vi "GPS PositionChange Event Example.vi"() -> ()   [LabVIEW 2012, in "Phidget GPS.lvlib"]
uses:
  <instrlib>/Phidgets/Phidget GPS/Phidget GPS.lvlib
  <instrlib>/Phidgets/Phidget GPS/Public/GPSStart.vi
  <instrlib>/Phidgets/Phidget GPS/Public/GPSClose.vi
  <instrlib>/Phidgets/Phidget Common/Phidget Common.lvlib
panel:
  out "Latitude":dbl
  out "Longitude":dbl
  out "Altitude":dbl
  in  "stop":bool
  out "Serial Number Return":i32
  in  "Device Info":T1={"Serial Number"=-1, "Channel"=0, "Port"=0}
  out "error out":errorcluster
  # "Be sure to use this stop button to stop the program.\nIf you use the \"Abort Execution\" button, you will\nneed to use PhidgetResetLibrary.vi or restart Labview \nin order for any Phidgets to work."
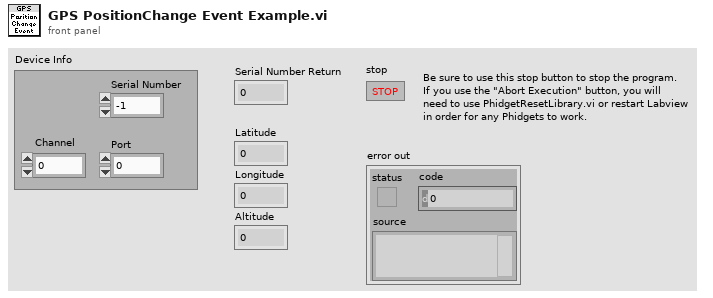
[diagram p1: front panel]
types:
  T1 = cluster{"Serial Number":i32, "Channel":i32, "Port":i32}
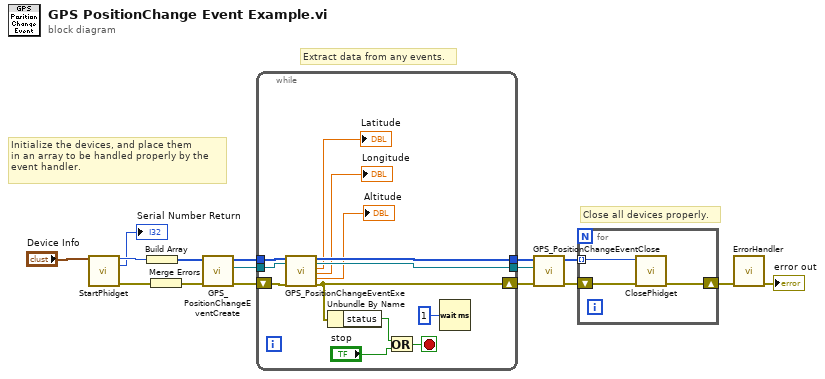
[diagram p0: block diagram]
diagram:
  # "Close all devices properly."
  # "Extract data from any events."
  # "Initialize the devices, and place them\nin an array to be handled properly by the\nevent handler."
  n1 = call-poly <instrlib>:"StartPhidget.vi"("Device Info"="Device Info") -> ("Phidget ID"=w5:u64, "Serial Number Return"=→"Serial Number Return":i32, "error out"=w1:errorcluster)  [unwired: 11 in, 1 out]
  n2 = Build Array(w5) -> (w16:u64[])
  n3 = Merge Errors(w1) -> (w7:errorcluster)
  n4 = call <instrlib>:"GPS_PositionChangeEventCreate.vi"("error in (no error)"=w7, "Devices In"=w16) -> ("error out"=w9:errorcluster, "Event Registration Refnum"=w14:refnum<event-registration>, "Devices Out"=w15:u64[])  [unwired: 7 in]
  n5 = while {
    tunnel: w15 -> [w29]
    tunnel: w14 -> [w24]
    tunnel: [w28] -> w11
    shift-right: [w23] -> w10
    shift-left: w9 -> [w27]
    tunnel: [w25] -> w3
    stop <- w22 stop-if-true
    n6 = call <instrlib>:"GPS_PositionChangeEventExe.vi"("Devices In"=w29, "Event Registration Refnum In"=w24, "error in (no error)"=w27) -> ("Devices Out"=w25:u64[], "Event Registration Refnum Out"=w28:refnum<event-registration>, "Latitude"=→"Latitude":dbl, "Longitude"=→"Longitude":dbl, "Altitude"=→"Altitude":dbl, "error out"=w23:errorcluster)  [unwired: 8 in, 3 out]
    n7 = Unbundle By Name(w23) -> ("status"=w20:bool)
    n8 = Or(x=w20, y="stop") -> (x .or. y?=w22:bool)
    n9 = Wait (ms)(milliseconds to wait=u32 1) -> ()  [unwired: 1 out]
  }
  n10 = call <instrlib>:"GPS_PositionChangeEventClose.vi"("error in (no error)"=w10, "Event Registration Refnum In"=w11, "Devices In"=w3) -> ("error out"=w6:errorcluster, "Devices Out"=w4:u64[])  [unwired: 7 in]
  n11 = for {
    tunnel: w4 -> [w30] mode=indexing
    shift-right: [w32] -> w13
    shift-left: w6 -> [w31]
    n12 = call-poly <instrlib>:"ClosePhidget.vi"("error in"=w31, "Device In"=w30) -> ("error out"=w32:errorcluster)  [unwired: 9 in]
  }
  n13 = call <instrlib>:"ErrorHandler.vi"("error in"=w13) -> ("error out"=→"error out":errorcluster)  [unwired: 9 in, 1 out]
